vi "Check if position is correcct.vi"(8 "error in (no error)":errorcluster, 10 "Tolerance (um)":dbl, 11 "Tomo in":refnum<class "Tomo.lvclass">) -> (0 "error out":errorcluster, 2 "correct?":bool, 3 "Tomo out":refnum<class "Tomo.lvclass">)   [LabVIEW 2012, in "Tomo.lvclass"]
uses:
  Tomo.lvclass
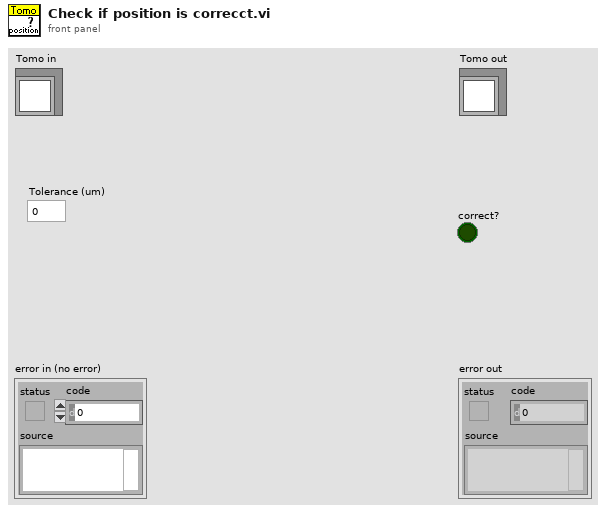
[diagram p1: front panel]
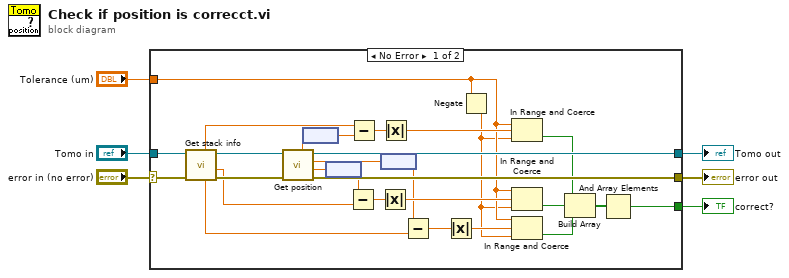
[diagram p0: block diagram]
diagram:
  n1 = case shown="No Error" "error in (no error)" {
    selector: "error in (no error)" -> [w33 w36]
    tunnel: [w31 w36] -> w5
    tunnel: [w29 w35] -> w3
    tunnel: "Tomo in" -> [w34 w35]
    tunnel: "Tolerance (um)" -> [w13 _]
    tunnel: [w7 _] -> w1
    frame No Error {
      n2 = call-dynamic "Get stack info.vi"("error in (no error)"=w33, "Tomo in"=w34) -> ("error out"=w32:errorcluster, "Z start"=w16:dbl, "Tomo out"=w30:refnum<class "Tomo.lvclass">, "Y position"=w15:dbl, "X position"=w19:dbl)  [unwired: 4 in, 1 out]
      n3 = call-dynamic "Get position.vi"("error in (no error)"=w32, "Tomo in"=w30) -> ("error out"=w31:errorcluster, "Z position"=w26:dbl[unit], "Y position"=w24:dbl[unit], "Tomo out"=w29:refnum<class "Tomo.lvclass">, "X position"=w28:dbl[unit])  [unwired: 4 in, 1 out]
      n4 = node(w28) -> (w18:dbl)
      n5 = node(w26) -> (w17:dbl)
      n6 = Subtract(x=w17, y=w16) -> (x-y=w25:dbl)
      n7 = Subtract(x=w19, y=w18) -> (x-y=w27:dbl)
      n8 = Absolute Value(x=w25) -> (abs(x)=w21:dbl)
      n9 = Absolute Value(x=w27) -> (abs(x)=w20:dbl)
      n10 = node(w24) -> (w14:dbl)
      n11 = Subtract(x=w14, y=w15) -> (x-y=w23:dbl)
      n12 = Absolute Value(x=w23) -> (abs(x)=w22:dbl)
      n13 = Negate(x=w13) -> (-x=w12:dbl)
      n14 = In Range and Coerce(upper limit=w13, x=w20, lower limit=w12) -> (In Range?=w11:bool)  [unwired: 1 out]
      n15 = In Range and Coerce(upper limit=w13, x=w21, lower limit=w12) -> (In Range?=w10:bool)  [unwired: 1 out]
      n16 = In Range and Coerce(upper limit=w13, x=w22, lower limit=w12) -> (In Range?=w9:bool)  [unwired: 1 out]
      n17 = Build Array(w11, w10, w9) -> (w8:bool[])
      n18 = And Array Elements(Boolean array=w8) -> (logical AND=w7:bool)
    }
    frame Error {
    }
  }
  "error out" <- w5
  "Tomo out" <- w3
  "correct?" <- w1
